vi "CorrectErrors.vi"(8 "Error In":errorcluster, 11 "Encoded Data":u8[](array[numeric])) -> (0 "Error Out":errorcluster, 2 "Success":bool, 3 "Corrected Data":u8[](array[numeric]))   [LabVIEW 2010]
uses:
  RScode.dll
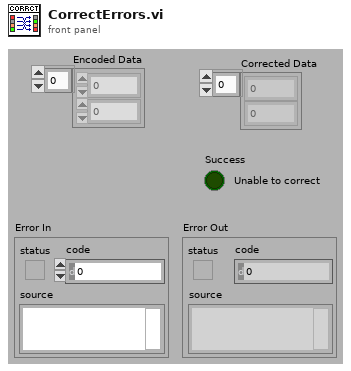
[diagram p1: front panel]
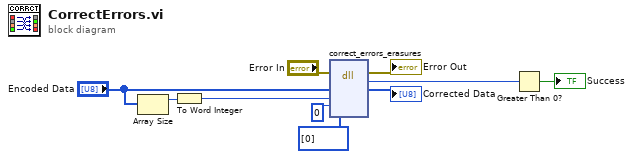
[diagram p0: block diagram]
diagram:
  n1 = Array Size(array="Encoded Data") -> (size(s)=w10:i32)
  n2 = To Word Integer(number=w10) -> (16bit integer=w5:i16)
  n3 = dll-call lib="Z:/Ted On My Mac/GitHub/Configurator/Source/Utilities/RScode/RScode.dll" fn="correct_errors_erasures"(error in="Error In", "codeword"="Encoded Data", "csize"=w5, "nerasures"=i16 0, "interasures"=i16[] [0]) -> (error out=→"Error Out":errorcluster, "return type"=w2:i16, "codeword"=→"Corrected Data":u8[])  [unwired: 5 in, 1 out]
  n4 = Greater Than 0?(x=w2) -> (x > 0?=→"Success":bool)
